vi "Get Actor Data.vi"(8 "error in (no error)":errorcluster, 10 "Actor's Self Q":refnum<class "Message Enqueuer.lvclass">, 11 "Monitor Data in":refnum<class "Monitor Data.lvclass">) -> (0 "error out":errorcluster, 1 "Nested Actors":refnum<class "Message Enqueuer.lvclass">[](array[class]), 2 "Actor Data":T1={"Actor Type"="", "Actor Cores"=[], "Self"=refnum, "Caller"=refnum, "Actor Label"="", "Last Ping"=-1.0}, 4 "Found?":bool)   [LabVIEW 2017, in "MGI-Monitored Actor Core.lvlib" / "Monitor Data.lvclass"]
doc: "Returns information about the specified actor\n\nCopyright: MGI 2016\nAuthor: Derek Trepanier"
uses:
  Monitor Data.lvclass
  <vilib>/ActorFramework/Message Enqueuer/Message Enqueuer.lvclass
  Actor Data.ctl
  Monitor Data.lvclass/Monitor Data.ctl
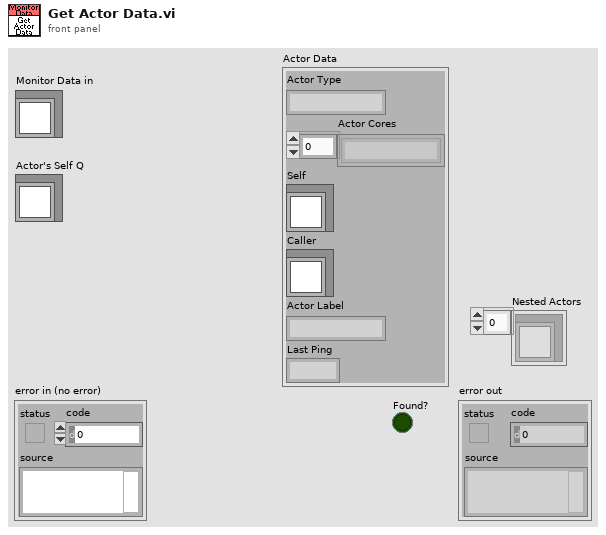
[diagram p1: front panel]
types:
  T1 = typedef "MGI-Monitored Actor Core.lvlib/Monitor Data.lvclass/Actor Data.ctl" = cluster{"Actor Type":string, "Actor Cores":string[], "Self":refnum<class "Message Enqueuer.lvclass">, "Caller":refnum<class "Message Enqueuer.lvclass">, "Actor Label":string, "Last Ping":dbl}
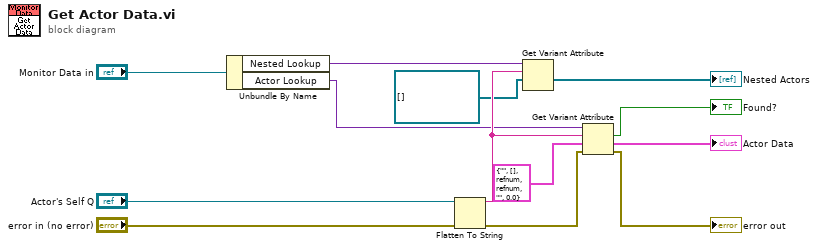
[diagram p0: block diagram]
diagram:
  n1 = Unbundle By Name("Monitor Data in") -> ("Nested Lookup"=w2:variant, "Actor Lookup"=w1:variant)
  n2 = Flatten To String(anything="Actor's Self Q", error in (no error)="error in (no error)") -> (data string=w4:string, error out=w5:errorcluster)  [unwired: 2 in, 1 out]
  n3 = Get Variant Attribute(Variant=w2, name=w4, default value (empty Variant)=refnum<class "Message Enqueuer.lvclass">[] []) -> (value=→"Nested Actors":refnum<class "Message Enqueuer.lvclass">[])  [unwired: 1 in, 3 out]
  n4 = Get Variant Attribute(Variant=w1, name=w4, default value (empty Variant)=T1 {"Actor Type"="", "Actor Cores"=[], "Self"=refnum, "Caller"=refnum, "Actor Label"="", "Last Ping"=0.0} ("Actor Data"), error in=w5) -> (found=→"Found?":bool, value=→"Actor Data":T1, error out=→"error out":errorcluster)  [unwired: 1 out]
